vi "Add Helper Library To Project.vi"(8 "error in":errorcluster, 9 "New Library Name":string, 10 "Library Path":path, 11 "Project ref":refnum<vi>) -> (0 "error out":errorcluster)   [LabVIEW 2020, in "MeasurementService Editor.lvlib"]
uses:
  MeasurementService Editor.lvlib
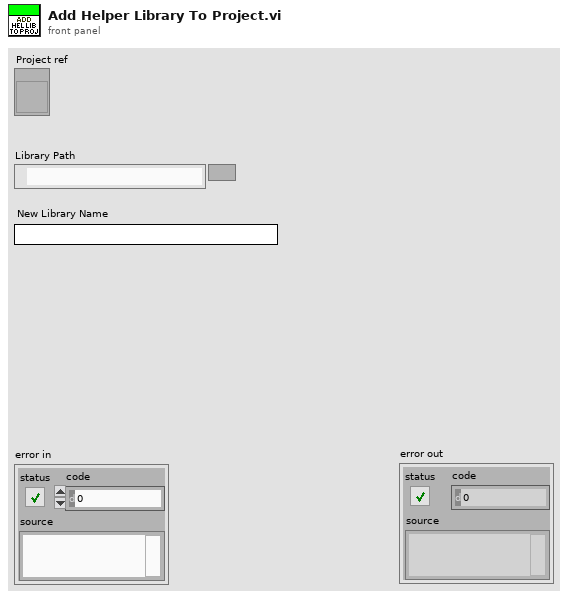
[diagram p1: front panel]
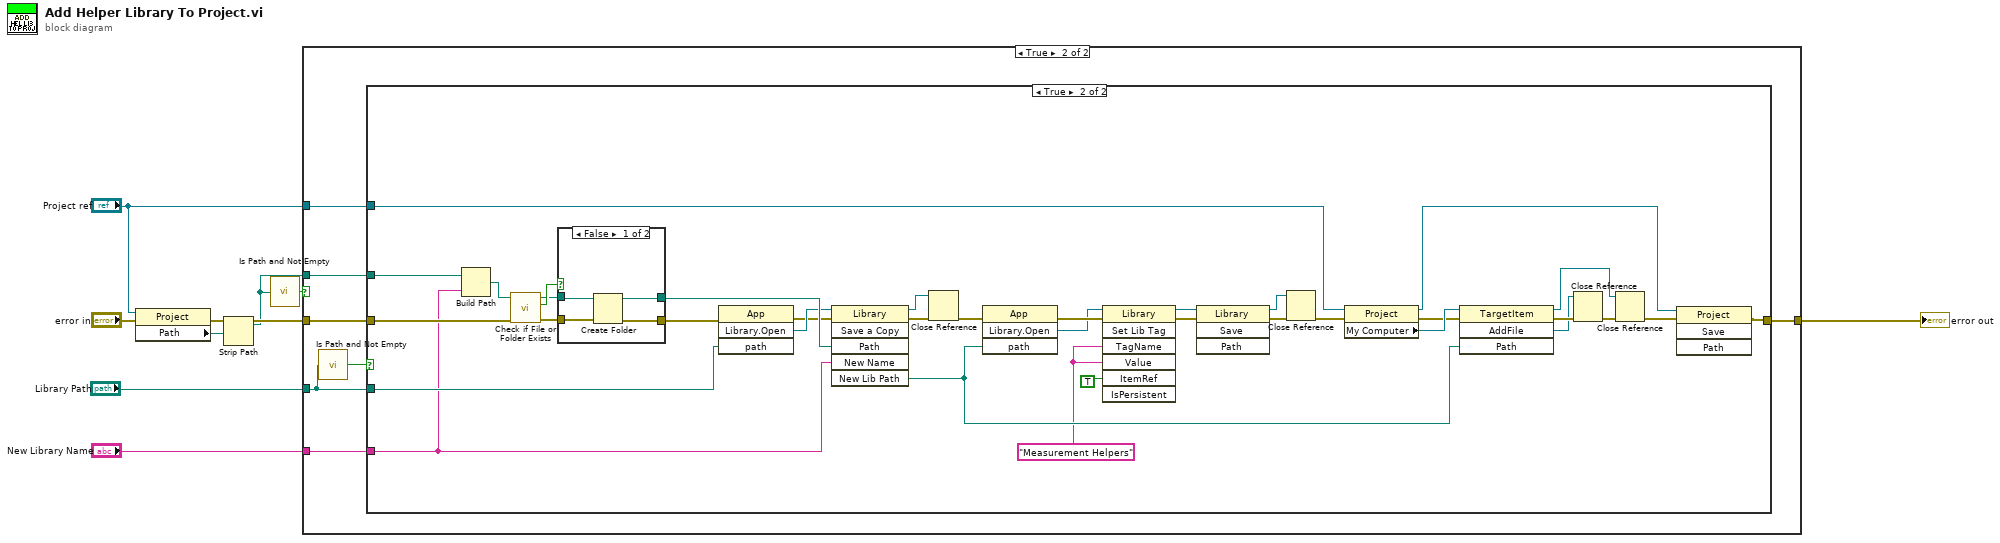
[diagram p0: block diagram]
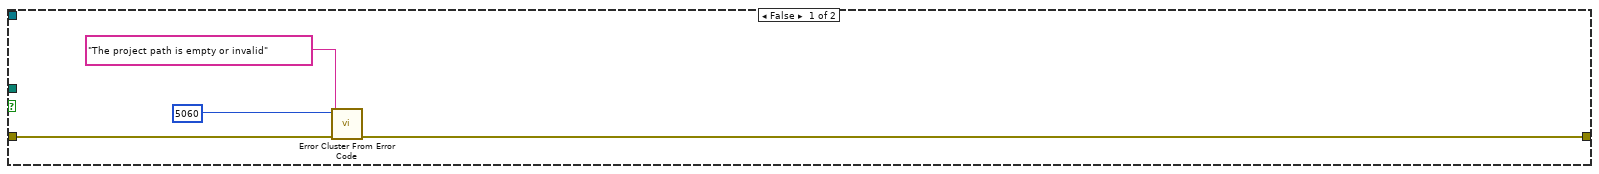
[diagram p2: hidden frame]
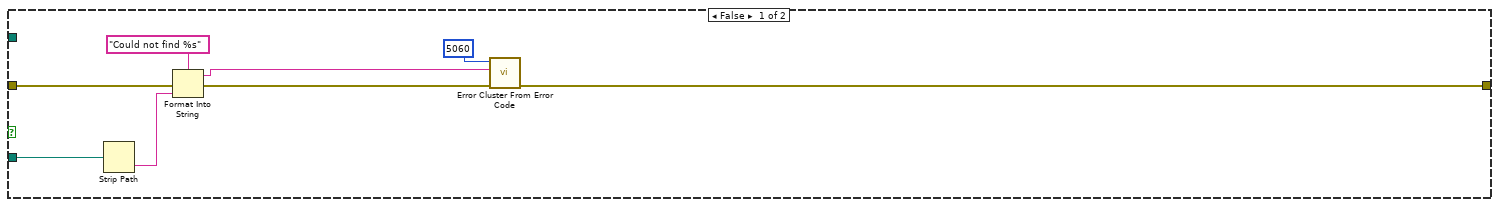
[diagram p3: hidden frame]
diagram:
  n1 = property class="Project"(reference="Project ref", error in="error in") -> (error out=w6:errorcluster, "Path"=w3:path)  [unwired: 1 out]
  n2 = Strip Path(path=w3) -> (stripped path=w2:path)  [unwired: 1 out]
  n3 = call <vilib>:"Is Path and Not Empty.vi"("path"=w2) -> ("Is Path and Not Empty?"=w9:bool)  [unwired: 4 in]
  n4 = case shown="True" w9 {
    tunnel: w6 -> [w13 w20]
    tunnel: [w12 w19] -> w8
    tunnel: "Library Path" -> [_ w17]
    tunnel: "New Library Name" -> [_ w16]
    tunnel: w2 -> [_ w15]
    tunnel: "Project ref" -> [_ w14]
    frame False {
      n5 = call <vilib>:"Error Cluster From Error Code.vi"("error in (no error)"=w13, "error message (\"\")"="The project path is empty or invalid" ("error message (\"\")"), "error code (0)"=5060) -> ("error out"=w12:errorcluster)  [unwired: 6 in]
    }
    frame True {
      n6 = call <vilib>:"Is Path and Not Empty.vi"("path"=w17) -> ("Is Path and Not Empty?"=w18:bool)  [unwired: 4 in]
      n7 = case shown="True" w18 {
        tunnel: w20 -> [w27 w63]
        tunnel: [w26 w61] -> w19
        tunnel: w17 -> [w23 w62]
        tunnel: w16 -> [_ w52]
        tunnel: w15 -> [_ w60]
        tunnel: w14 -> [_ w59]
        frame False {
          n8 = Strip Path(path=w23) -> (name=w24:string)  [unwired: 1 out]
          n9 = Format Into String(format string="Could not find %s", error in=w27, w24) -> (resulting string=w21:string, error out=w25:errorcluster)  [unwired: 1 in]
          n10 = call <vilib>:"Error Cluster From Error Code.vi"("error in (no error)"=w25, "error message (\"\")"=w21, "error code (0)"=5060) -> ("error out"=w26:errorcluster)  [unwired: 6 in]
        }
        frame True {
          w31 = "Measurement Helpers" ("Tag Name")
          n11 = Build Path(base path=w60, name or relative path=w52) -> (appended path=w58:path)
          n12 = call <vilib>:"Check if File or Folder Exists.vi"("error in (no error)"=w63, "path"=w58) -> ("error out"=w55:errorcluster, "file or folder exists?"=w57:bool, "dup path"=w56:path)  [unwired: 7 in]
          n13 = case shown="False" w57 {
            tunnel: w56 -> [w66 w69]
            tunnel: w55 -> [w67 w68]
            tunnel: [w65 w68] -> w54
            tunnel: [w64 w69] -> w53
            frame False {
              n14 = Create Folder(path (use dialog)=w66, error in=w67) -> (created path=w64:path, error out=w65:errorcluster)  [unwired: 1 in, 1 out]
            }
            frame True {
            }
          }
          n15 = invoke class="App" method="Library.Open"(error in=w54, "path"=w62) -> (error out=w38:errorcluster, "Open Library"=w51:refnum<vi>)  [unwired: 2 in, 2 out]
          n16 = invoke class="Library" method="Save a Copy"(reference=w51, error in=w38, "Path"=w53, "New Name"=w52) -> (reference out=w46:refnum<vi>, error out=w48:errorcluster, "New Lib Path"=w37:path)  [unwired: 2 in, 3 out]
          n17 = Close Reference(reference=w46, error in (no error)=w48) -> (error out=w47:errorcluster)
          n18 = invoke class="App" method="Library.Open"(error in=w47, "path"=w37) -> (error out=w45:errorcluster, "Open Library"=w32:refnum<vi>)  [unwired: 2 in, 2 out]
          n19 = invoke class="Library" method="Set Lib Tag"(reference=w32, error in=w45, "TagName"=w31, "Value"=w31, "ItemRef"=TRUE ("Is Persistent")) -> (reference out=w29:refnum<vi>, error out=w33:errorcluster)  [unwired: 2 in, 5 out]
          n20 = invoke class="Library" method="Save"(reference=w29, error in=w33) -> (reference out=w43:refnum<vi>, error out=w44:errorcluster)  [unwired: 2 in, 2 out]
          n21 = Close Reference(reference=w43, error in (no error)=w44) -> (error out=w42:errorcluster)
          n22 = property class="Project"(reference=w59, error in=w42) -> (reference out=w39:refnum<vi>, error out=w49:errorcluster, "My Computer"=w50:refnum<vi>)
          n23 = invoke class="TargetItem" method="AddFile"(reference=w50, error in=w49, "Path"=w37) -> (reference out=w34:refnum<vi>, error out=w41:errorcluster, "AddFile"=w40:refnum<vi>)  [unwired: 1 in, 1 out]
          n24 = Close Reference(reference=w40, error in (no error)=w41) -> (error out=w36:errorcluster)
          n25 = Close Reference(reference=w34, error in (no error)=w36) -> (error out=w35:errorcluster)
          n26 = invoke class="Project" method="Save"(reference=w39, error in=w35) -> (error out=w61:errorcluster)  [unwired: 2 in, 3 out]
        }
      }
    }
  }
  "error out" <- w8
